vi "Clusterwitharraystring.vi"(1 "Cluster In":cluster{"Array In":string[], "String":string}, 2 "String To Append":string) -> (0 "Cluster Out":cluster{"Array Out":string[], "String":string})   [LabVIEW 2012]
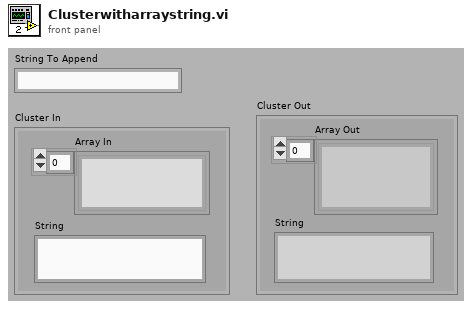
[diagram p1: front panel]
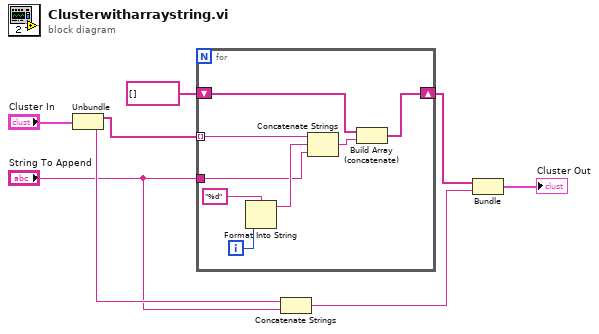
[diagram p0: block diagram]
diagram:
  n1 = Unbundle("Cluster In") -> ("Array In"=w6:string[], "String"=w5:string)
  n2 = for {
    tunnel: w6 -> [w16] mode=indexing
    shift-right: [w13] -> w2
    shift-left: string[] [] -> [w14]
    tunnel: "String To Append" -> [w10]
    i -> [w12]
    n3 = Format Into String(format string="%d", w12) -> (resulting string=w11:string)  [unwired: 2 in, 1 out]
    n4 = Concatenate Strings(w16, w11, w10) -> (w15:string)
    n5 = Build Array (concatenate)(w14, w15) -> (w13:string[])
  }
  n6 = Concatenate Strings(w5, "String To Append") -> (w1:string)
  n7 = Bundle(w2, w1) -> (→"Cluster Out":cluster{string[], string})  [unwired: 1 out]
